vi "Get or Set Control Panel Values.vi"(7 "Actions":T1, 10 "Flattened String [In]":string, 11 "This VI":refnum<vi>) -> (2 "Flattened String [Out]":string)   [LabVIEW 2014]
uses:
  Controls/FGV Actions.ctl
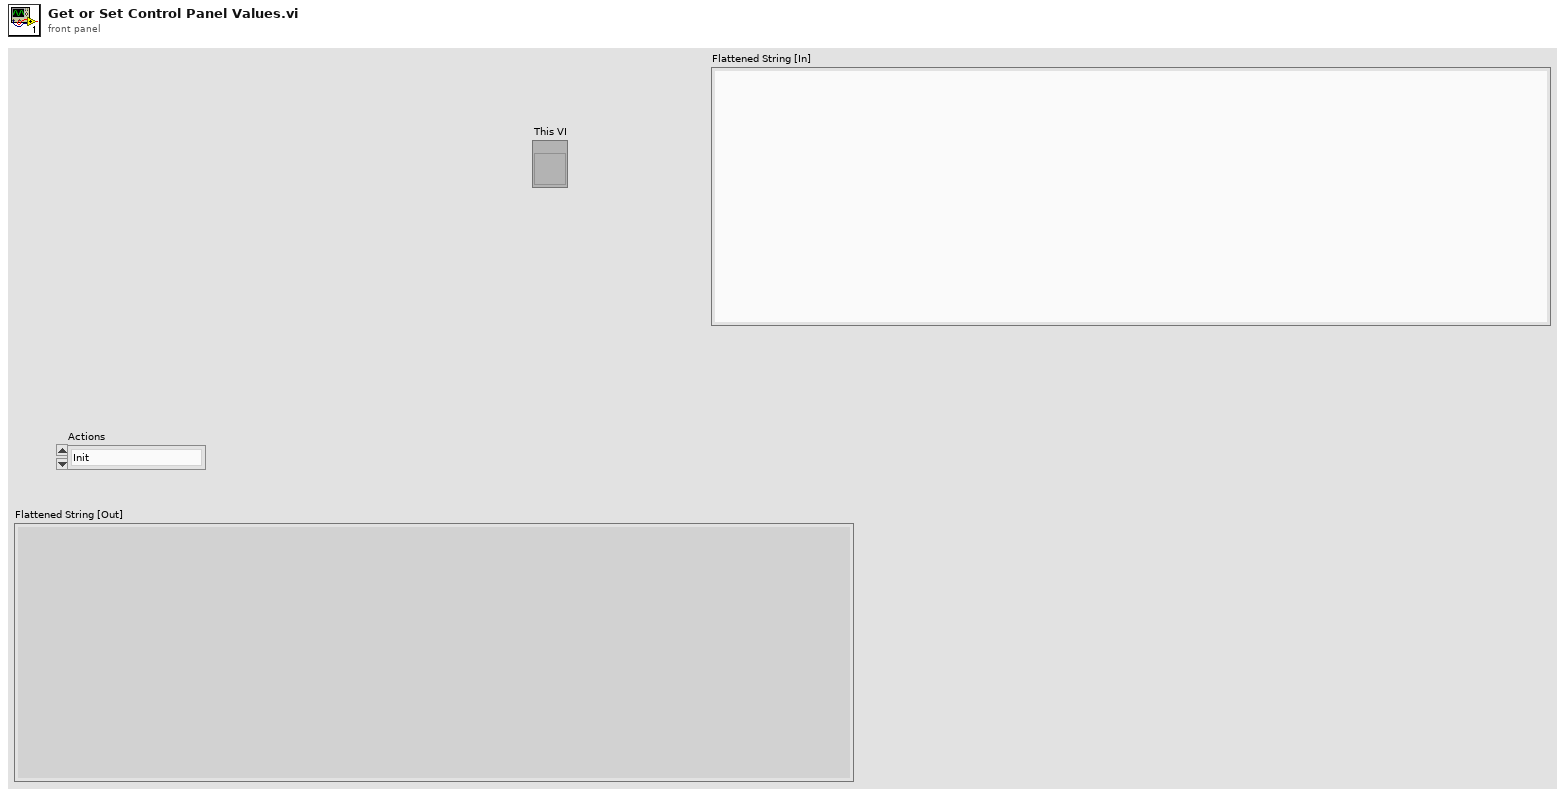
[diagram p1: front panel]
types:
  T1 = typedef "FGV Actions.ctl" = enum16{"Init", "Set", "Get", "Clear"}
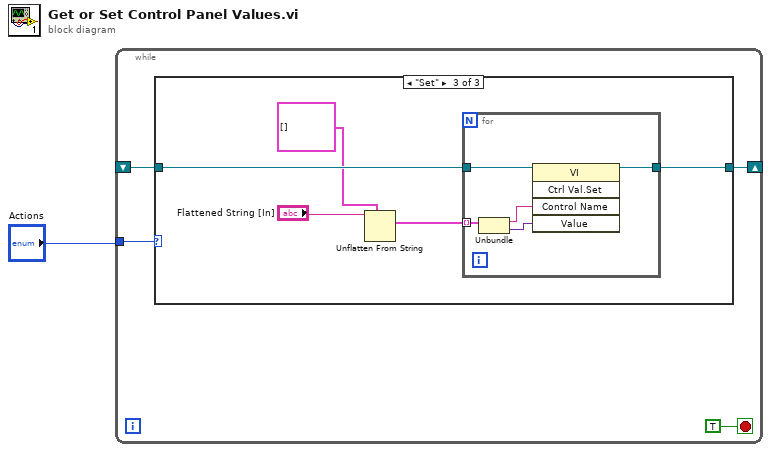
[diagram p0: block diagram]
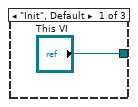
[diagram p2: hidden frame]
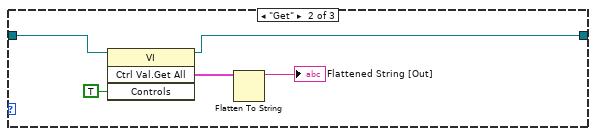
[diagram p3: hidden frame]
diagram:
  n1 = while {
    shift-right: [w4] -> _
    shift-left: _ -> [w3]
    tunnel: "Actions" -> [w5]
    stop <- TRUE stop-if-true
    n2 = case shown="\"Set\"" w5 {
      tunnel: ["This VI" w9 w15] -> w4
      tunnel: w3 -> [_ w10 w16]
      frame "Init", Default {
      }
      frame "Get" {
        n3 = invoke class="VI" method="Ctrl Val.Get All"(reference=w10, "Controls"=TRUE) -> (reference out=w9:refnum<vi>, "Get All Control Values Variant"=w8:cluster{"Name":string, "Variant Data":variant}[])  [unwired: 2 in, 2 out]
        n4 = Flatten To String(anything=w8) -> (data string=→"Flattened String [Out]":string)  [unwired: 3 in, 2 out]
      }
      frame "Set" {
        n5 = Unflatten From String(type=cluster{"Name":string, "Variant Data":variant}[] [] ("Control Value:Get All"), binary string="Flattened String [In]") -> (value=w12:cluster{"Name":string, "Variant Data":variant}[])  [unwired: 3 in, 2 out]
        n6 = for {
          tunnel: w16 -> [w21]
          tunnel: [w20] -> w15
          tunnel: w12 -> [w19] mode=indexing
          n7 = Unbundle(w19) -> ("Name"=w18:string, "Variant Data"=w17:variant)
          n8 = invoke class="VI" method="Ctrl Val.Set"(reference=w21, "Control Name"=w18, "Value"=w17) -> (reference out=w20:refnum<vi>)  [unwired: 2 in, 4 out]
        }
      }
    }
  }
